vi "AI data read single.vi"(8 "error in (no error)":errorcluster, 10 "Numeric":i32, 11 "Message Queues in":T1) -> (0 "error out":errorcluster, 3 "Array":dbl[](array[numeric]))   [LabVIEW 2014]
uses:
  support/Message Queue/All Message Queues.ctl
  support/Message Queue/Message Cluster.ctl
  support/Message Queue/Enqueue Message (Single).vi
  support/Message Queue/Message Queue.lvlib
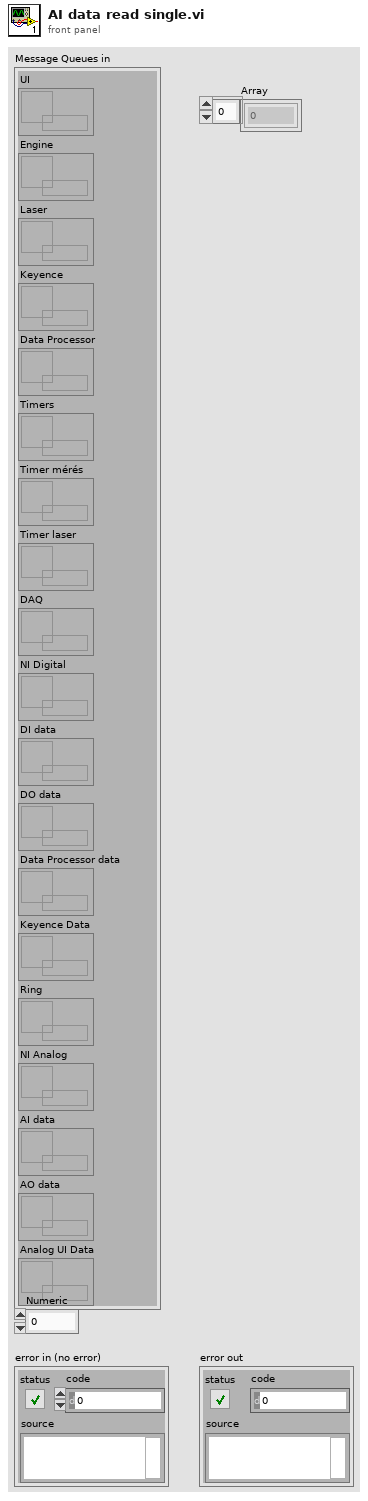
[diagram p1: front panel]
types:
  T1 = typedef "Message Queue.lvlib/All Message Queues.ctl" = cluster{"UI":refnum<queue>, "Engine":refnum<queue>, "Laser":refnum<queue>, "Keyence":refnum<queue>, "Data Processor":refnum<queue>, "Timers":refnum<queue>, "Timer mérés":refnum<queue>, "Timer laser":refnum<queue>, "DAQ":refnum<queue>, "NI Digital":refnum<queue>, "DI data":refnum<queue>, "DO data":refnum<queue>, "Data Processor data":refnum<queue>, "Keyence Data":refnum<queue>, "Ring":refnum<queue>, "NI Analog":refnum<queue>, "AI data":refnum<queue>, "AO data":refnum<queue>, "Analog UI Data":refnum<queue>}
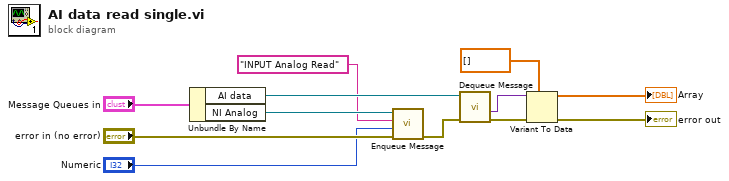
[diagram p0: block diagram]
diagram:
  n1 = Unbundle By Name("Message Queues in") -> ("AI data"=w10:refnum<queue>, "NI Analog"=w5:refnum<queue>)
  n2 = call-poly "Enqueue Message.vi"("error in (no error)"="error in (no error)", "Message Data"="Numeric", "Message"="INPUT Analog Read", "Message Queue"=w5) -> ("error out"=w8:errorcluster)  [unwired: 6 in, 1 out]
  n3 = call "Dequeue Message.vi"("error in (no error)"=w8, "Message Queue"=w10) -> ("error out"=w3:errorcluster, "Message Data"=w9:variant)  [unwired: 5 in, 3 out]
  n4 = Variant To Data(error in=w3, type=dbl[] [], Variant=w9) -> (data=→"Array":dbl[], error out=→"error out":errorcluster)
